vi "sg Query Clock Error.vi"(8 "error in (no error)":errorcluster, 10 "error":dbl, 11 "device":i32) -> (0 "error out":dbl, 2 "function return":u32(ring), 3 "error out 2":errorcluster)   [LabVIEW 2014, in "VSG25A.lvlib"]
doc: "SG_API sgStatus sgQueryClockError(int device, double *error);"
uses:
  VSG25A.lvlib
  sg_api.dll
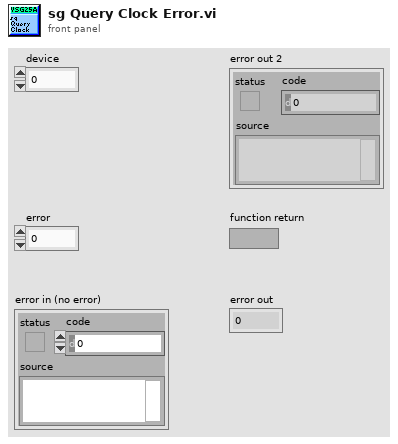
[diagram p1: front panel]
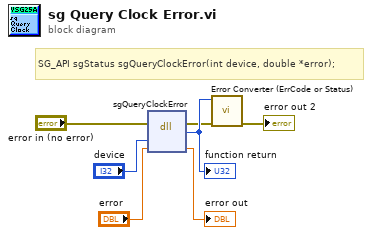
[diagram p0: block diagram]
diagram:
  # "SG_API sgStatus sgQueryClockError(int device, double *error);"
  n1 = dll-call lib="C:/Users/M_LAPTOP/Desktop/Labview/practice/VSG25A/sg_lib/sg_api.*" fn="sgQueryClockError"(error in="error in (no error)", "device"="device", "error"="error") -> (error out=w2:errorcluster, w7:u32, "error"=→"error out":dbl)  [unwired: 3 in, 1 out]
  "function return" <- w7
  n2 = call "Error Converter (ErrCode or Status).vi"("error in (no error)"=w2, "error code"=w7) -> ("error out"=→"error out 2":errorcluster)  [unwired: 9 in]
